vi "Configure Hardware.vi"(8 "error in (no error)":errorcluster, 11 "Hardware Resources in":T1={"Tasks"=[{"DAQmx Task"="Mod3AI0-Temp", "Read-Write Radio"=enum."Read"}, {"DAQmx Task"="Mod3AI0-Temp", "Read-Write Radio"=enum."Read"}]}) -> (0 "error out":errorcluster, 3 "Hardware Resources out":T1={"Tasks"=[{"DAQmx Task"="Mod3AI0-Temp", "Read-Write Radio"=enum."Read"}, {"DAQmx Task"="Mod3AI0-Temp", "Read-Write Radio"=enum."Read"}]})   [LabVIEW 2018, in "DAQ.lvlib"]
doc: "Configure the hardware."
uses:
  DAQ/DAQ.lvlib
  Hardware Configuration.ctl
  Task Cluster.ctl
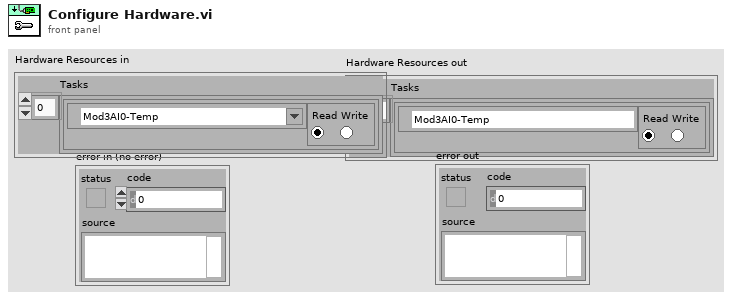
[diagram p1: front panel]
types:
  T1 = typedef "DAQ.lvlib/Hardware Configuration.ctl" = cluster{"Tasks":T2[]}
  T2 = typedef "Task Cluster.ctl" = cluster{"DAQmx Task":refnum<k21>, "Read-Write Radio":enum32{"Read", "Write"}}
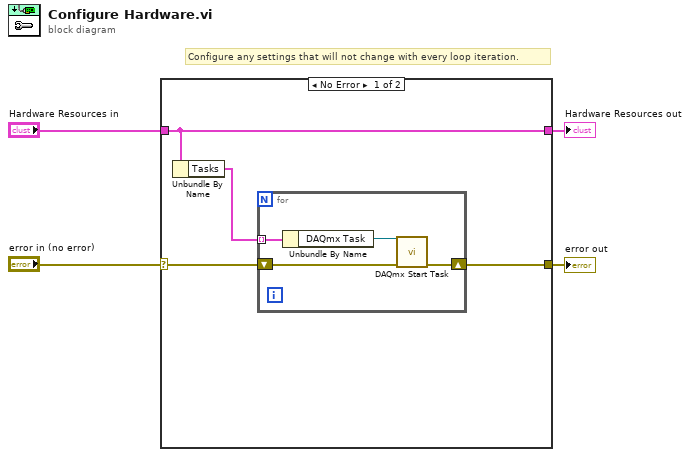
[diagram p0: block diagram]
diagram:
  # "Configure any settings that will not change with every loop iteration."
  n1 = case shown="No Error" "error in (no error)" {
    selector: "error in (no error)" -> [w5 w13]
    tunnel: [w7 w13] -> w3
    tunnel: "Hardware Resources in" -> [w8 w14]
    tunnel: [w8 w14] -> w1
    frame No Error {
      n2 = Unbundle By Name(w8) -> ("Tasks"=w6:T2[])
      n3 = for {
        tunnel: w6 -> [w9] mode=indexing
        shift-right: [w12] -> w7
        shift-left: w5 -> [w11]
        n4 = Unbundle By Name(w9) -> ("DAQmx Task"=w10:refnum<k21>)
        n5 = call <vilib>:"DAQmx Start Task.vi"("task/channels in"=w10, "error in"=w11) -> ("error out"=w12:errorcluster)  [unwired: 12 in, 1 out]
      }
    }
    frame Error {
    }
  }
  "Hardware Resources out" <- w1
  "error out" <- w3
